vi "F Dwf Digital I2c Write One.vi"(7 "pNak":i32, 8 "error in (no error)":errorcluster, 9 "bTx":u8, 10 "adr8bits":u8, 11 "hdwf":i32) -> (0 "error out":errorcluster, 3 "function return":i32, 5 "pNak out":i32)   [LabVIEW 2021, in "Olasdwf.lvlib"]
doc: "DWFAPI int FDwfDigitalI2cWriteOne(HDWF hdwf, unsigned char adr8bits, unsigned char bTx, int *pNak);"
uses:
  Olasdwf.lvlib
  Windows/System32/dwf.dll
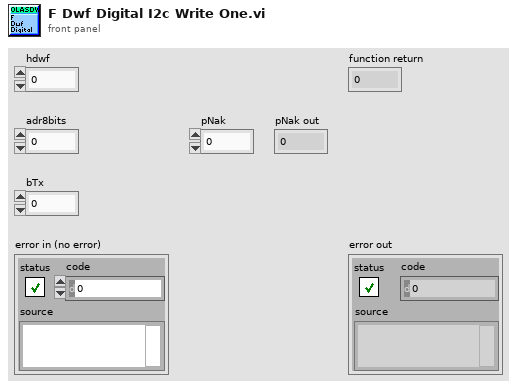
[diagram p1: front panel]
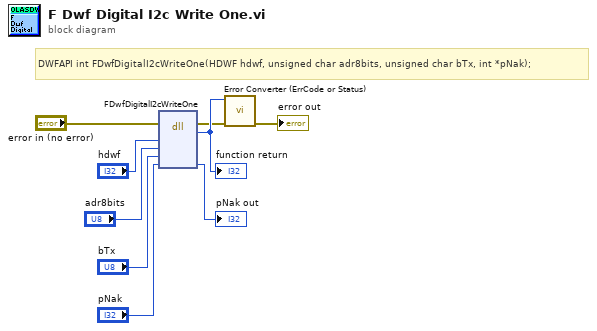
[diagram p0: block diagram]
diagram:
  # "DWFAPI int FDwfDigitalI2cWriteOne(HDWF hdwf, unsigned char adr8bits, unsigned char bTx, int *pNak);"
  n1 = dll-call lib="/Windows/System32/dwf.*" fn="FDwfDigitalI2cWriteOne"(error in="error in (no error)", "hdwf"="hdwf", "adr8bits"="adr8bits", "bTx"="bTx", "pNak"="pNak") -> (error out=w2:errorcluster, w9:i32, "pNak"=→"pNak out":i32)  [unwired: 5 in, 1 out]
  "function return" <- w9
  n2 = call "Error Converter (ErrCode or Status).vi"("error in (no error)"=w2, "error code"=w9) -> ("error out"=→"error out":errorcluster)  [unwired: 9 in]
